vi "set_list_content.vi"(8 "error in":errorcluster, 9 "Type":T1[](array[typedef]), 10 "Contents":string[](array[string]), 11 "matFile_info IN":T2) -> (0 "error out":errorcluster, 2 "Contents":string[](array[string]), 3 "matFile_info OUT":T2)   [LabVIEW 2018]
uses:
  MatFile_information.ctl
  type_control.ctl
panel:
  out "concatenated string":string
  out "length":i32
  out "Numeric Control":i32
  out "name array dim":i32
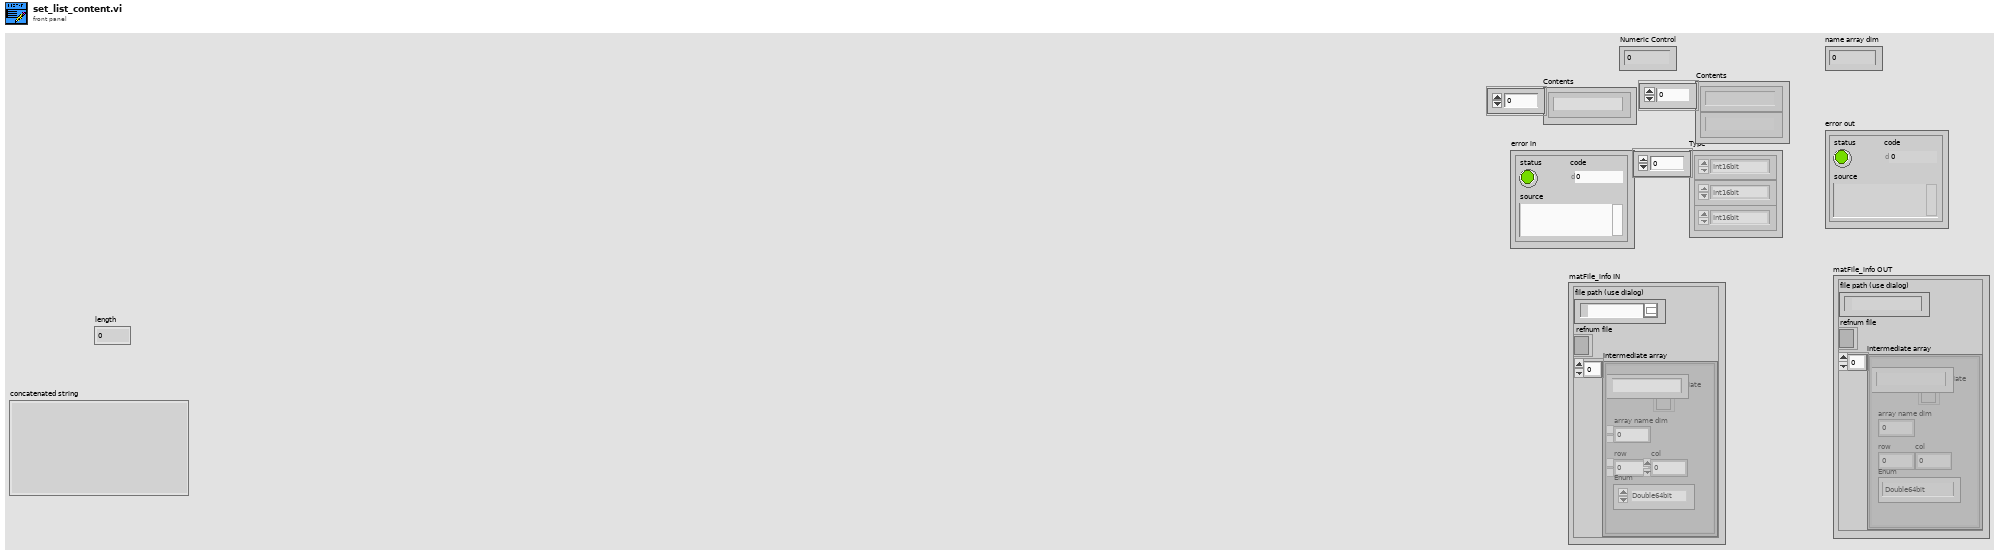
[diagram p1: front panel]
types:
  T1 = typedef "type_control.ctl" = enum16{"Int8bit_elem", "Int8bit", "Int64bit_elem", "Int64bit", "Int16bit_elem", "Double64bit_elem", "Int16bit", "Double64bit"}
  T2 = typedef "MatFile_information.ctl" = cluster{"file path (use dialog)":path, "refnum file":refnum<file>, "intermediate array":cluster{"intermediate":refnum<file>, "array name dim":i32, "row":i32, "col":i32, "Content":string, "Enum":T1}[]}
  T3 = cluster{"intermediate":refnum<file>, "array name dim":i32, "row":i32, "col":i32, "Content":string, "Enum":T1}
  T4 = enum16{"open", "replace", "create", "open or create", "replace or create", "replace or create with confirmation"}
  T5 = enum16{"big-endian, network order", "native, host order", "little-endian"}
  T6 = cluster{"miMATRIX":i32, "dimensione_content":i32, "miUINT32":i32, "n_byte flag":i32, "mxINT64_CLASS":i8, "undefined":i8, "I16":i16, "I32":i32, "miINT32":i32, i32, "row":i32, "col":i32, "miINT8":i32}
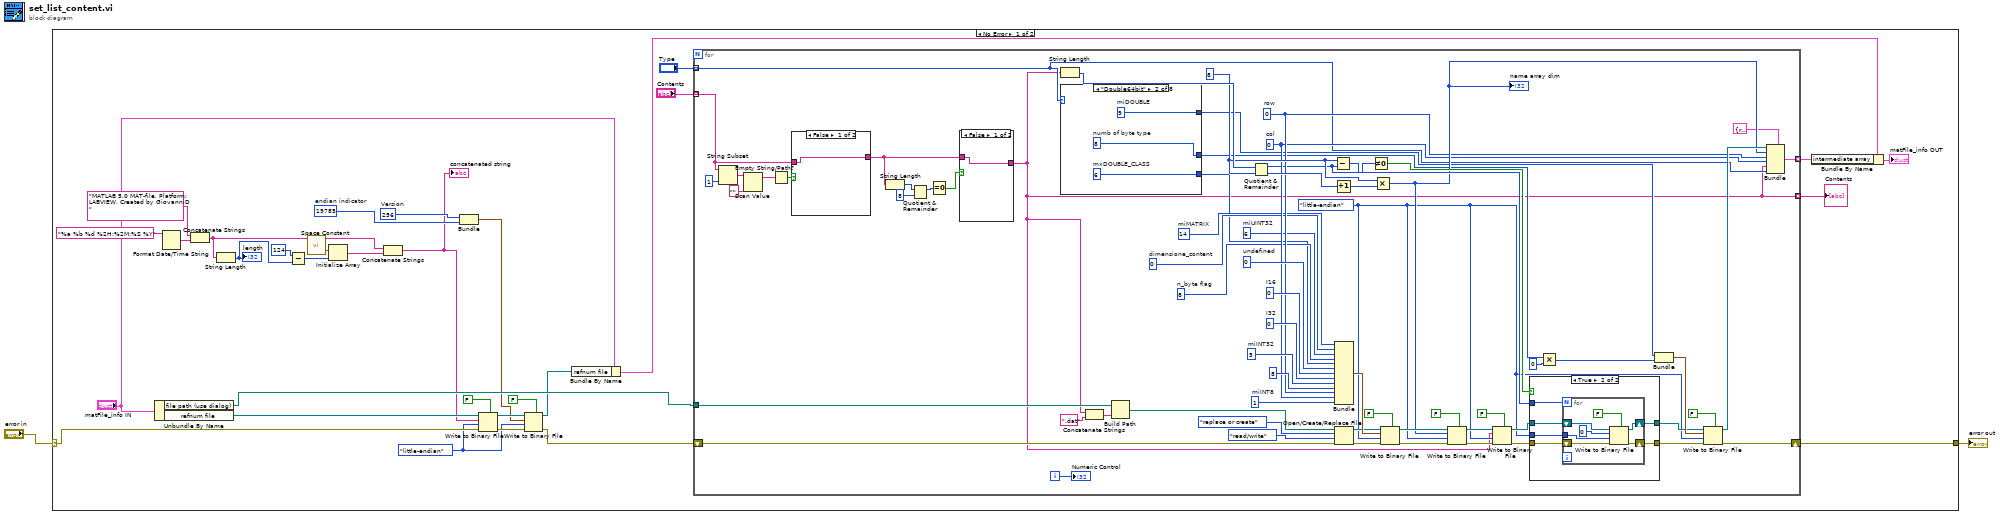
[diagram p0: block diagram]
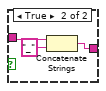
[diagram p2: hidden frame]
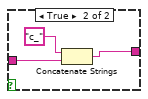
[diagram p3: hidden frame]
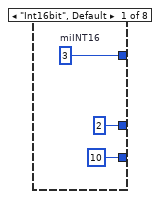
[diagram p4: hidden frame]
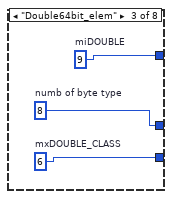
[diagram p5: hidden frame]
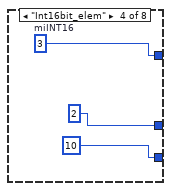
[diagram p6: hidden frame]
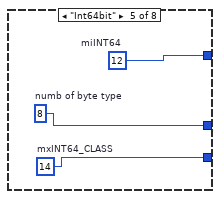
[diagram p7: hidden frame]
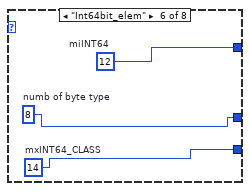
[diagram p8: hidden frame]
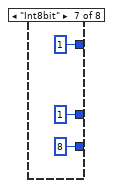
[diagram p9: hidden frame]
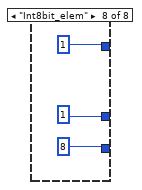
[diagram p10: hidden frame]
diagram:
  n1 = case shown="No Error" "error in" {
    selector: "error in" -> [w12 w148]
    tunnel: [w32 w148] -> w1
    frame No Error {
      w18 = i16 256  # Version
      w17 = i16 19785  # endian indicator
      w11 = T5."little-endian" ("byte order (0:big-endian, network order)")
      n2 = Unbundle By Name("matFile_info IN") -> ("file path (use dialog)"=w9:path, "refnum file"=w8:refnum<file>)
      n3 = Format Date/Time String(time format string (%c)="%a %b %d %2H:%2M:%S %Y") -> (date/time string=w25:string)  [unwired: 2 in]
      n4 = Concatenate Strings("MATLAB 5.0 MAT-file, Platform: LABVIEW, Created by GiovanniD ", w25) -> (w20:string)
      n5 = String Length(string=w20) -> (length=w23:i32)
      "length" <- w23
      n6 = Subtract(x=124, y=w23) -> (x-y=w21:i32)
      n7 = call <vilib>:"Space Constant.vi"() -> ("String"=w24:string)
      n8 = Initialize Array(w24, w21) -> (w19:string[])
      n9 = Concatenate Strings(w20, w19) -> (w7:string)
      "concatenated string" <- w7
      n10 = Bundle("Version"=w18, "endian indicator"=w17) -> (w6:cluster{"Version":i16, "endian indicator ":i16})  [unwired: 1 in]
      n11 = Write to Binary File(file (use dialog)=w8, data=w7, error in=w12, 5:FALSE ("prepend array or string size? (T)"), 9:w11) -> (refnum out=w15:refnum<file>, error out=w16:errorcluster)  [unwired: 1 in, 1 out]
      n12 = Write to Binary File(file (use dialog)=w15, data=w6, error in=w16, 5:FALSE ("prepend array or string size? (T)"), 9:w11) -> (refnum out=w3:refnum<file>, error out=w10:errorcluster)  [unwired: 1 in, 1 out]
      n13 = Bundle By Name(cluster="matFile_info IN", "refnum file"=w3) -> (w4:T2)
      n14 = for {
        tunnel: "Contents" -> [w40] mode=indexing
        tunnel: w9 -> [w100]
        shift-right: [w98] -> w32
        shift-left: w10 -> [w99]
        tunnel: [w97] -> w31 mode=indexing
        tunnel: "Type" -> [w47] mode=indexing
        tunnel: [w34] -> w28 mode=indexing
        i -> [w46]
        w51 = T5."little-endian" ("byte order (0:big-endian, network order)")
        w78 = 8 ("y")
        w85 = 1  # miINT8
        w68 = 0  # col
        w69 = 0  # row
        w88 = 5  # miINT32
        w89 = 0  # I32
        w90 = i16 0  # I16
        w91 = i8 0  # undefined
        w59 = 8  # n_byte flag
        w60 = 6  # miUINT32
        w61 = 0  # dimensione_content
        w62 = 14  # miMATRIX
        n15 = String Subset(string=w40, length (rest)=1 ("length (rest)")) -> (substring=w44:string)  [unwired: 1 in]
        n16 = Scan Value(string=w44, format string="") -> (output string=w45:string)  [unwired: 1 in, 1 out]
        n17 = Empty String/Path?(string/path=w45) -> (empty?=w41:bool)
        n18 = case shown="False" w41 {
          tunnel: w40 -> [w105 w107]
          tunnel: [w105 w106] -> w35
          frame False {
          }
          frame True {
            n19 = Concatenate Strings("c_", w107) -> (w106:string)
          }
        }
        n20 = String Length(string=w35) -> (length=w39:i32)
        n21 = Quotient & Remainder(x=w39, y=8) -> (x-y*floor(x/y)=w37:i32)  [unwired: 1 out]
        n22 = Equal To 0?(x=w37) -> (x = 0?=w36:bool)
        n23 = case shown="False" w36 {
          tunnel: w35 -> [w101 w104]
          tunnel: [w101 w102] -> w34
          frame False {
          }
          frame True {
            n24 = Concatenate Strings(w104, "_" ("string")) -> (w102:string)
          }
        }
        n25 = String Length(string=w34) -> (length=w84:i32)
        n26 = case shown="\"Double64bit\"" w47 {
          tunnel: [i8 10 ("mxDOUBLE_CLASS") w114 w115 i8 10 ("mxDOUBLE_CLASS") w121 w124 i8 8 ("mxINT64_CLASS") i8 8 ("mxINT64_CLASS")] -> w50
          tunnel: [w110 w113 w117 w120 w123 w126 1 ("miINT64") 1 ("miINT64")] -> w49
          tunnel: [2 ("numb of byte type") w112 w116 2 ("numb of byte type") w122 w125 1 ("numb of byte type") 1 ("numb of byte type")] -> w48
          frame "Int16bit", Default {
            w110 = 3  # miINT16
          }
          frame "Double64bit" {
            w112 = 8  # numb of byte type
            w113 = 9  # miDOUBLE
            w114 = i8 6  # mxDOUBLE_CLASS
          }
          frame "Double64bit_elem" {
            w116 = 8  # numb of byte type
            w117 = 9  # miDOUBLE
            w115 = i8 6  # mxDOUBLE_CLASS
          }
          frame "Int16bit_elem" {
            w120 = 3  # miINT16
          }
          frame "Int64bit" {
            w121 = i8 14  # mxINT64_CLASS
            w122 = 8  # numb of byte type
            w123 = 12  # miINT64
          }
          frame "Int64bit_elem" {
            w124 = i8 14  # mxINT64_CLASS
            w125 = 8  # numb of byte type
            w126 = 12  # miINT64
          }
          frame "Int8bit" {
          }
          frame "Int8bit_elem" {
          }
        }
        n27 = Concatenate Strings(w34, ".dat" ("element")) -> (w95:string)
        n28 = Build Path(base path=w100, name or relative path=w95) -> (appended path=w94:path)
        n29 = Quotient & Remainder(x=w84, y=w78) -> (x-y*floor(x/y)=w63:i32, floor(x/y)=w83:i32)
        n30 = Subtract(x=w78, y=w63) -> (x-y=w77:i32)
        n31 = Increment(x=w83) -> (x+1=w82:i32)
        n32 = Bundle("miMATRIX"=w62, "dimensione_content"=w61, "miUINT32"=w60, "n_byte flag"=w59, "mxINT64_CLASS"=w50, "undefined"=w91, "I16"=w90, "I32"=w89, "miINT32"=w88, 8, "row"=w69, "col"=w68, "miINT8"=w85) -> (w86:T6)  [unwired: 1 in]
        n33 = Open/Create/Replace File(file path (use dialog)=w94, error in=w99, operation (0:open)=T4."replace or create", access (0:read/write)=enum16{"read/write", "read-only", "write-only"}."read/write") -> (refnum out=w53:refnum<file>, error out=w52:errorcluster)  [unwired: 2 in, 1 out]
        n34 = Not Equal To 0?(x=w63) -> (x != 0?=w79:bool)
        n35 = Multiply(x=w78, y=w82) -> (x*y=w70:i32)
        "name array dim" <- w70
        n36 = Write to Binary File(file (use dialog)=w53, data=w86, error in=w52, 5:FALSE ("prepend array or string size? (T)"), 9:w51) -> (refnum out=w81:refnum<file>, error out=w80:errorcluster)  [unwired: 1 in, 1 out]
        n37 = Write to Binary File(file (use dialog)=w81, data=w70, error in=w80, 5:FALSE ("prepend array or string size? (T)"), 9:w51) -> (refnum out=w54:refnum<file>, error out=w57:errorcluster)  [unwired: 1 in, 1 out]
        n38 = Write to Binary File(file (use dialog)=w54, data=w34, error in=w57, 5:FALSE ("prepend array or string size? (T)"), 9:w51) -> (refnum out=w55:refnum<file>, error out=w56:errorcluster)  [unwired: 1 in, 1 out]
        n39 = case shown="True" w79 {
          tunnel: w56 -> [w134 w139]
          tunnel: w77 -> [_ w135]
          tunnel: w55 -> [w133 w140]
          tunnel: [w133 w138] -> w72
          tunnel: [w134 w137] -> w73
          tunnel: w51 -> [_ w136]
          frame False {
          }
          frame True {
            n40 = for {
              N: w135 -> [_]
              tunnel: w136 -> [w143]
              shift-right: [w145] -> w138
              shift-left: w140 -> [w147]
              shift-right: [w144] -> w137
              shift-left: w139 -> [w146]
              n41 = Write to Binary File(file (use dialog)=w147, data=i8 0, error in=w146, 5:FALSE ("prepend array or string size? (T)"), 9:w143) -> (refnum out=w145:refnum<file>, error out=w144:errorcluster)  [unwired: 1 in, 1 out]
            }
          }
        }
        n42 = Multiply(x=w48, y=0) -> (x*y=w75:i32)
        n43 = Bundle("miINT64"=w49, w75) -> (w74:cluster{"miINT64":i32, i32})  [unwired: 1 in]
        n44 = Write to Binary File(file (use dialog)=w72, data=w74, error in=w73, 5:FALSE ("prepend array or string size? (T)"), 9:w51) -> (refnum out=w71:refnum<file>, error out=w98:errorcluster)  [unwired: 1 in, 1 out]
        n45 = Bundle(cluster=T3 {"intermediate"=refnum, "array name dim"=0, "row"=0, "col"=0, "Content"="", "Enum"=enum."Int16bit"} ("Cluster"), "intermediate"=w71, "array name dim"=w70, "row"=w69, "col"=w68, "Content"=w34, "Enum"=w47) -> (w97:T3)
        "Numeric Control" <- w46
      }
      "Contents" <- w28
      n46 = Bundle By Name(cluster=w4, "intermediate array"=w31) -> (→"matFile_info OUT":T2)
    }
    frame Error {
    }
  }
  "error out" <- w1
